vi "niRFUtil MEAS Max Measurement Bandwidth.vi"(8 "Meas2 Bandwidth (Hz)":dbl, 9 "Meas2 Sampling Rate (Hz)":dbl, 10 "Meas1 Bandwidth (Hz)":dbl, 11 "Meas1 Sampling Rate (Hz)":dbl) -> (3 "Max Measurement Bandwidth (Hz)":dbl)   [LabVIEW 2015, in "niRFUtil.lvlib"]
uses:
  niRFUtil.lvlib
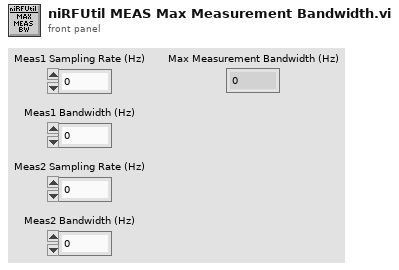
[diagram p1: front panel]
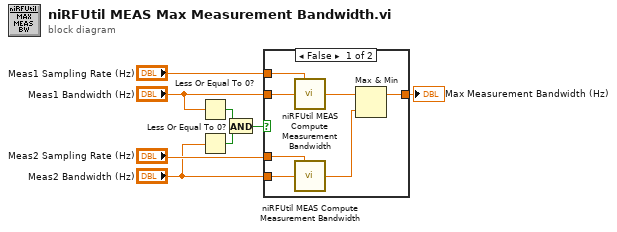
[diagram p0: block diagram]
diagram:
  n1 = Less Or Equal To 0?(x="Meas1 Bandwidth (Hz)") -> (x <= 0?=w2:bool)
  n2 = Less Or Equal To 0?(x="Meas2 Bandwidth (Hz)") -> (x <= 0?=w1:bool)
  n3 = And(x=w2, y=w1) -> (x .and. y?=w3:bool)
  n4 = case shown="False" w3 {
    tunnel: [w15 w16] -> w8
    tunnel: "Meas2 Sampling Rate (Hz)" -> [w13 _]
    tunnel: "Meas1 Sampling Rate (Hz)" -> [w11 _]
    tunnel: "Meas1 Bandwidth (Hz)" -> [w10 w16]
    tunnel: "Meas2 Bandwidth (Hz)" -> [w9 _]
    frame False {
      n5 = call "niRFUtil MEAS Compute Measurement Bandwidth.vi"("Sampling Rate (Hz)"=w11, "Meas Recommended BW (Hz)"=w10) -> ("Computed Meas BW (Hz)"=w12:dbl)  [unwired: 13 in]
      n6 = call "niRFUtil MEAS Compute Measurement Bandwidth.vi"("Sampling Rate (Hz)"=w13, "Meas Recommended BW (Hz)"=w9) -> ("Computed Meas BW (Hz)"=w14:dbl)  [unwired: 13 in]
      n7 = Max & Min(x=w12, y=w14) -> (max(x,y)=w15:dbl)  [unwired: 1 out]
    }
    frame True {
    }
  }
  "Max Measurement Bandwidth (Hz)" <- w8
